vi "Standard Engine.vi"(8 "error in":errorcluster, 9 "status notifier":refnum<notifier>, 10 "rt fifo":refnum<k33>, 11 "Engine Data":T1={"Main Tag Data"={"Double"=[], "Single"=[], "I64"=[], "I32"=[], "I16"=[], "I8"=[], "U64"=[], "U32"=[], "U16"=[], "U8"=[], "Boolean"=[], "String"=[], "Array of Double"=[], "Array of Single"=[], "Array of I64"=[], "Array of I32"=[], "Array of I16"=[], "Array of I8"=[], "Array of U64"=[], "Array of U32"=[], "Array of U16"=[], "Array of U8"=[], "Array of Boolean"=[], "Array of String"=[]}, "Module Info"={"Tag Bus Modules"=[], "Input Method Indices"=[], "Process Method Indices"=[], "Output Method Indices"=[], "Input Transfer Specifications"=[], "Parameter Transfer Specifications"=[], "Result Transfer Specifications"=[], "Output Transfer Specifications"=[], "Module Errors"=[], "UID"=""}, "Safe State?"=FALSE, "engine timing source"=refnum, "Processor"=-2, "Priority"=1, "dT"=0}) -> (0 "error out":errorcluster)   [LabVIEW 2013, in "synchronous engine runtime.lvclass"]
uses:
  synchronous engine runtime.lvclass
  Engine Data.ctl
  <vilib>/NI/Module Timing Source/timing source/TBM timing source.lvclass
  <vilib>/NI/Tag Bus/table/data table.ctl
  Module Execution Info.ctl
  <vilib>/NI/Tag Bus Module Framework/runtime/TBM module execution interface.lvclass
  Data Table with Transfer Spec.ctl
  <vilib>/NI/Tag Bus/table/transfer specification.ctl
  <vilib>/NI/Tag Bus/tag/Data Type.ctl
  Commands.ctl
  notifier.ctl
  Engine Runtime/Execution States.ctl
  <vilib>/Platform/TimedLoop/XDataNode/timing_clust.ctl
  <vilib>/Platform/TimedLoop/XDataNode/nitl_modes.ctl
  <vilib>/Platform/TimedLoop/XDataNode/wakeup.ctl
  <vilib>/NI/Tag Bus/table/transfer table data.vi
  <vilib>/Platform/TimedLoop/XDataNode/XDataNode.xnode
  Engine Runtime/Engine Runtime Interface.lvclass
  <vilib>/Platform/TimedLoop/XDataNode/XDNodeRunTimeDep.lvlib
  <vilib>/NI/Tag Bus/table/data table.lvlib
  <vilib>/NI/Tag Bus/tag/tag descriptor.lvclass
panel:
  out "iterations":i32
  in  "Network Address":string="10.1.128.117"
  in  "send trace?":bool
  out "loop period (ms)":u32
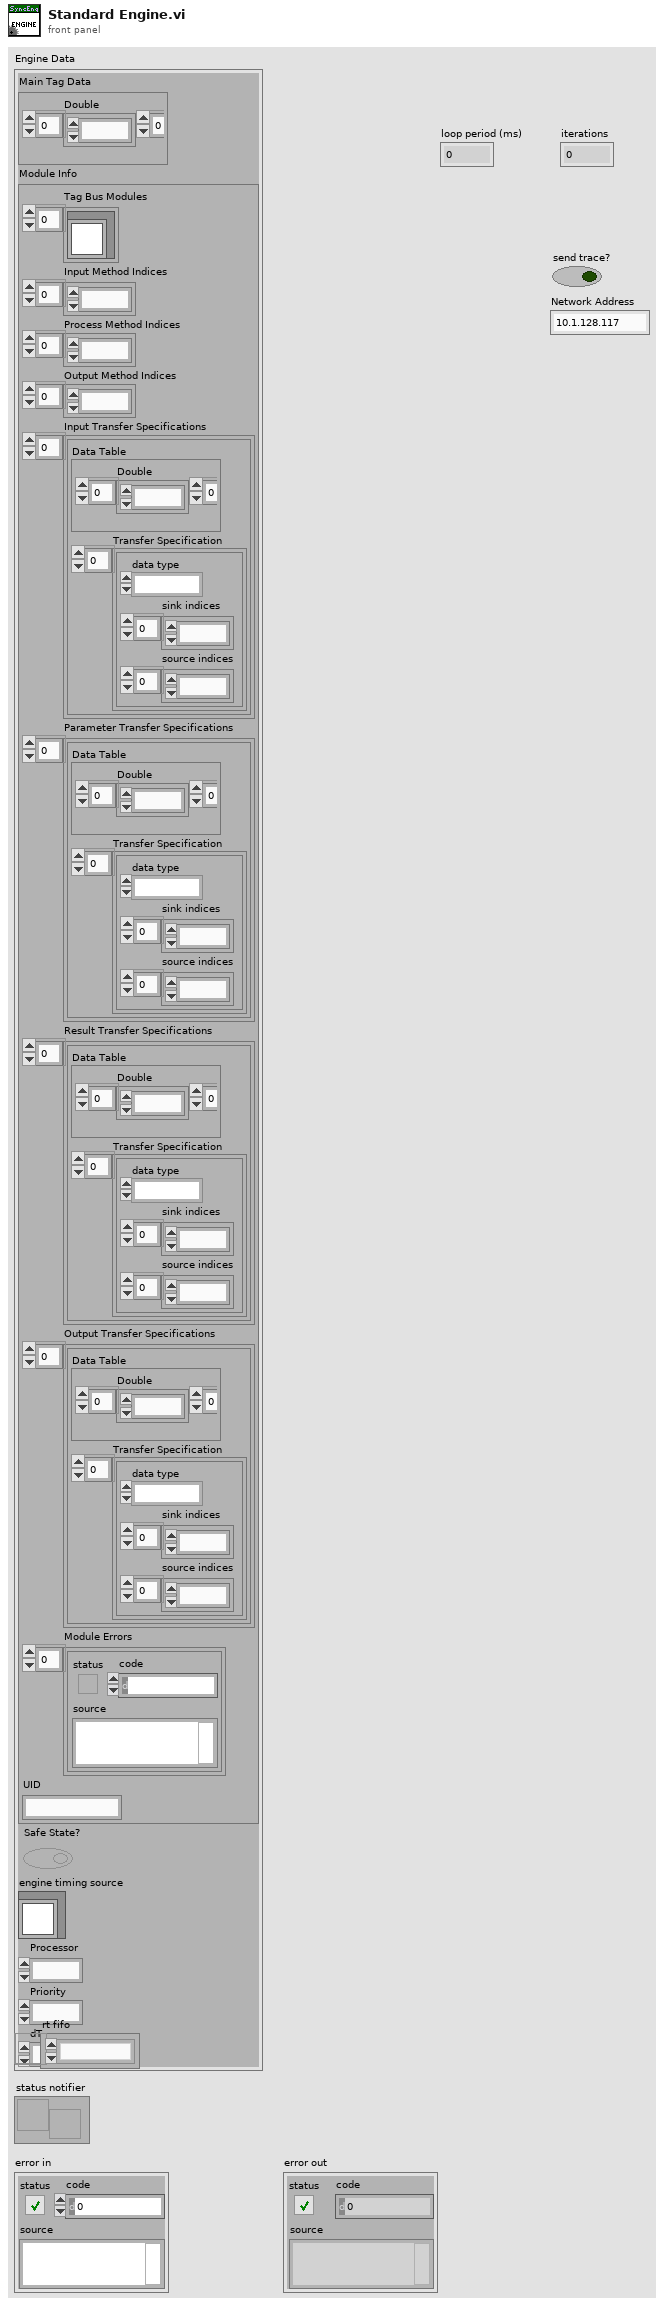
[diagram p1: front panel]
types:
  T1 = typedef "synchronous engine runtime.lvclass/Engine Data.ctl" = cluster{"Main Tag Data":T2, "Module Info":T3, "Safe State?":bool, "engine timing source":refnum<class "TBM timing source.lvclass">, "Processor":i32, "Priority":i32, "dT":u32}
  T2 = typedef "tag bus.lvlib/data table.lvlib/data table.ctl" = cluster{"Double":dbl[], "Single":sgl[], "I64":i64[], "I32":i32[], "I16":i16[], "I8":i8[], "U64":u64[], "U32":u32[], "U16":u16[], "U8":u8[], "Boolean":bool[], "String":string[], "Array of Double":cluster{"DBL Array":dbl[]}[], "Array of Single":cluster{"SGL Array":sgl[]}[], "Array of I64":cluster{"I64 Array":i64[]}[], "Array of I32":cluster{"I32 Array":i32[]}[], "Array of I16":cluster{"I16 Array":i16[]}[], "Array of I8":cluster{"I8 Array":i8[]}[], "Array of U64":cluster{"U64 Array":u64[]}[], "Array of U32":cluster{"U32 Array":u32[]}[], "Array of U16":cluster{"U16 Array":u16[]}[], "Array of U8":cluster{"U8 Array":u8[]}[], "Array of Boolean":cluster{"Boolean Array":bool[]}[], "Array of String":cluster{"String Array":string[]}[]}
  T3 = typedef "synchronous engine runtime.lvclass/Module Execution Info.ctl" = cluster{"Tag Bus Modules":refnum<class "TBM module execution interface.lvclass">[], "Input Method Indices":i32[], "Process Method Indices":i32[], "Output Method Indices":i32[], "Input Transfer Specifications":T4[], "Parameter Transfer Specifications":T4[], "Result Transfer Specifications":T4[], "Output Transfer Specifications":T4[], "Module Errors":errorcluster[], "UID":string}
  T4 = typedef "synchronous engine runtime.lvclass/Data Table with Transfer Spec.ctl" = cluster{"Data Table":T2, "Transfer Specification":T5[]}
  T5 = typedef "tag bus.lvlib/data table.lvlib/transfer specification.ctl" = cluster{"data type":T6, "sink indices":i32[], "source indices":i32[]}
  T6 = typedef "tag bus.lvlib/tag descriptor.lvclass/Data Type.ctl" = enum16{"Double", "Single", "I64", "I32", "I16", "I8", "U64", "U32", "U16", "U8", "Boolean", "String", "Array of Double", "Array of Single", "Array of I64", "Array of I32", "Array of I16", "Array of I8", "Array of U64", "Array of U32", "Array of U16", "Array of U8", "Array of Boolean", "Array of String"}
  T7 = typedef "Engine Runtime Interface.lvclass/Execution States.ctl" = enum16{"Initializing", "Paused (Initialized)", "Running", "Set Safe Outputs", "Uninitializing", "Stopped (Uninitialized)", "Error (Uninitialized)", "Safe State (Uninitialized)", "Closed"}
  T8 = typedef "synchronous engine runtime.lvclass/notifier.ctl" = cluster{"Engine State":T7, "error constant":errorcluster}
  T9 = typedef "synchronous engine runtime.lvclass/Commands.ctl" = enum16{"Start", "Pause", "Safe State", "Normal", "Stop", "Shutdown"}
  T10 = typedef "XDNodeRunTimeDep.lvlib/timing_clust.ctl" = cluster{"Expected End [f-1]":u64, "Actual End [f-1]":u64, "Finished Late? [f-1]":bool, "Expected End [i-1]":u64, "Actual End [i-1]":u64, "Finished Late? [i-1]":bool, "Expected Start [i]":u64, "Actual Start [i]":u64, "Expected Start [f]":u64, "Actual Start [f]":u64, "Source Name":string, "Structure Name":string, "Period":i64, "Deadline":i64, "Offset":i64, "Start":i64, "Priority":i32, "Timeout":i32, "Mode":T11, "Wakeup Reason":T12, "Error":errorcluster, "Source Type":string, "Secondary Source Type":string, "Global End Time":u64, "Global Start Time":u64, "Frame Duration":u64, "Iteration Duration":u64, "Assigned CPU":i32, "I/O Scan Engine Mode":u32}
  T11 = typedef "XDNodeRunTimeDep.lvlib/nitl_modes.ctl" = enum32{"No Change", "Process missed periods, maintain original phase", "Discard missed periods, maintain original phase", "Process missed periods, ignore original phase", "Discard missed periods, ignore original phase"}
  T12 = typedef "XDNodeRunTimeDep.lvlib/wakeup.ctl" = enum32{"Normal", "Aborted", "Asynchronous wakeup", "Timing source error", "Timed loop error", "Timeout"}
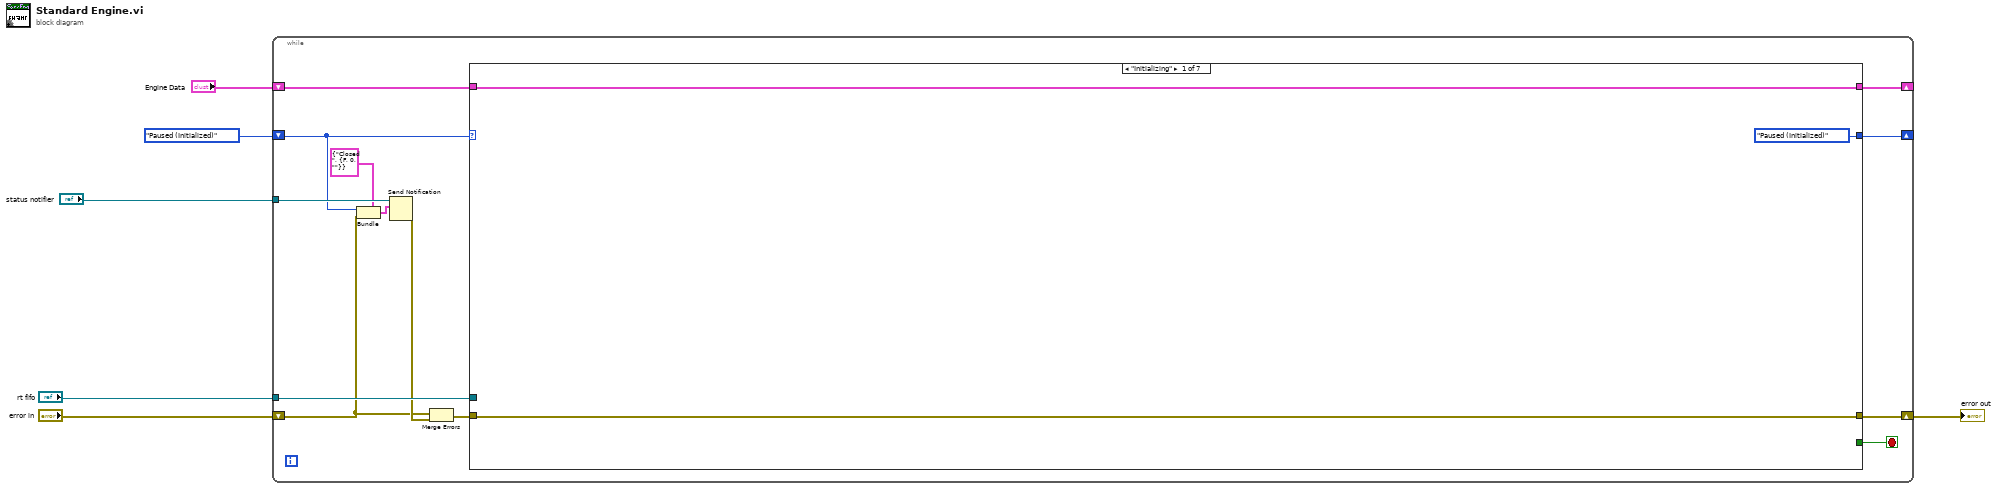
[diagram p0: block diagram]
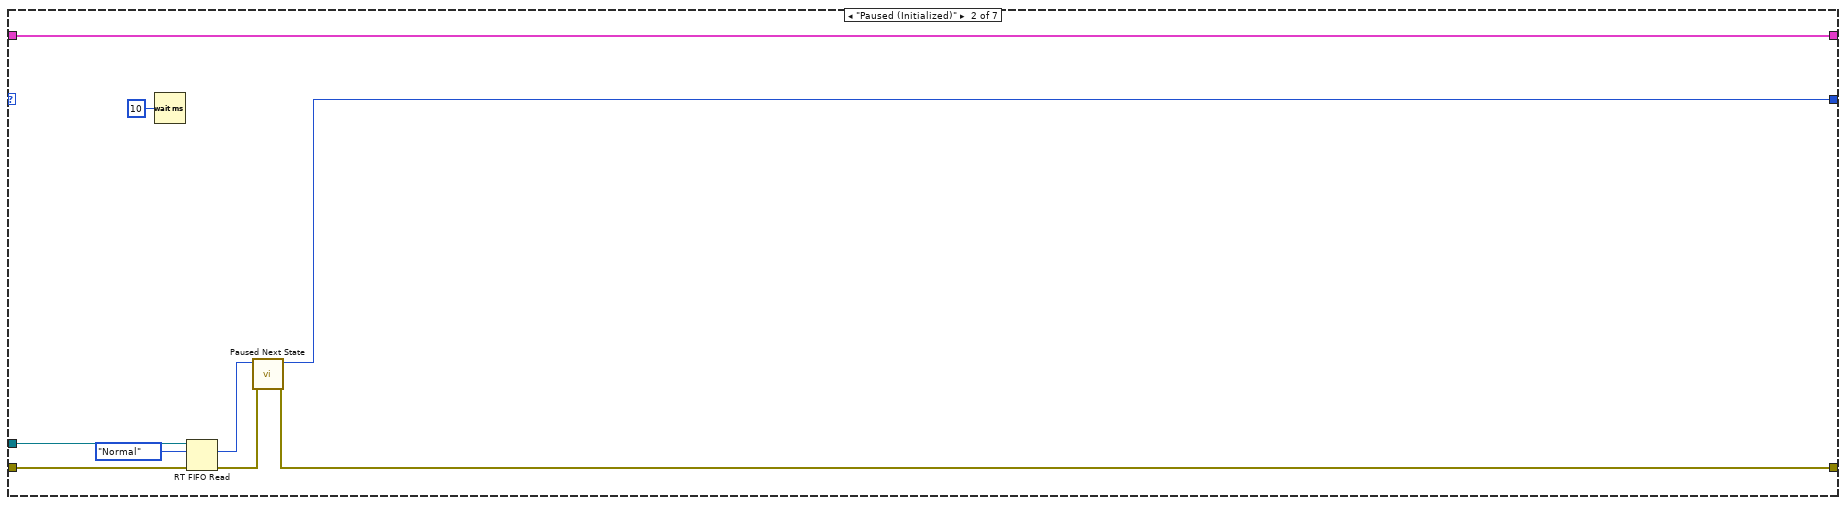
[diagram p2: hidden frame]
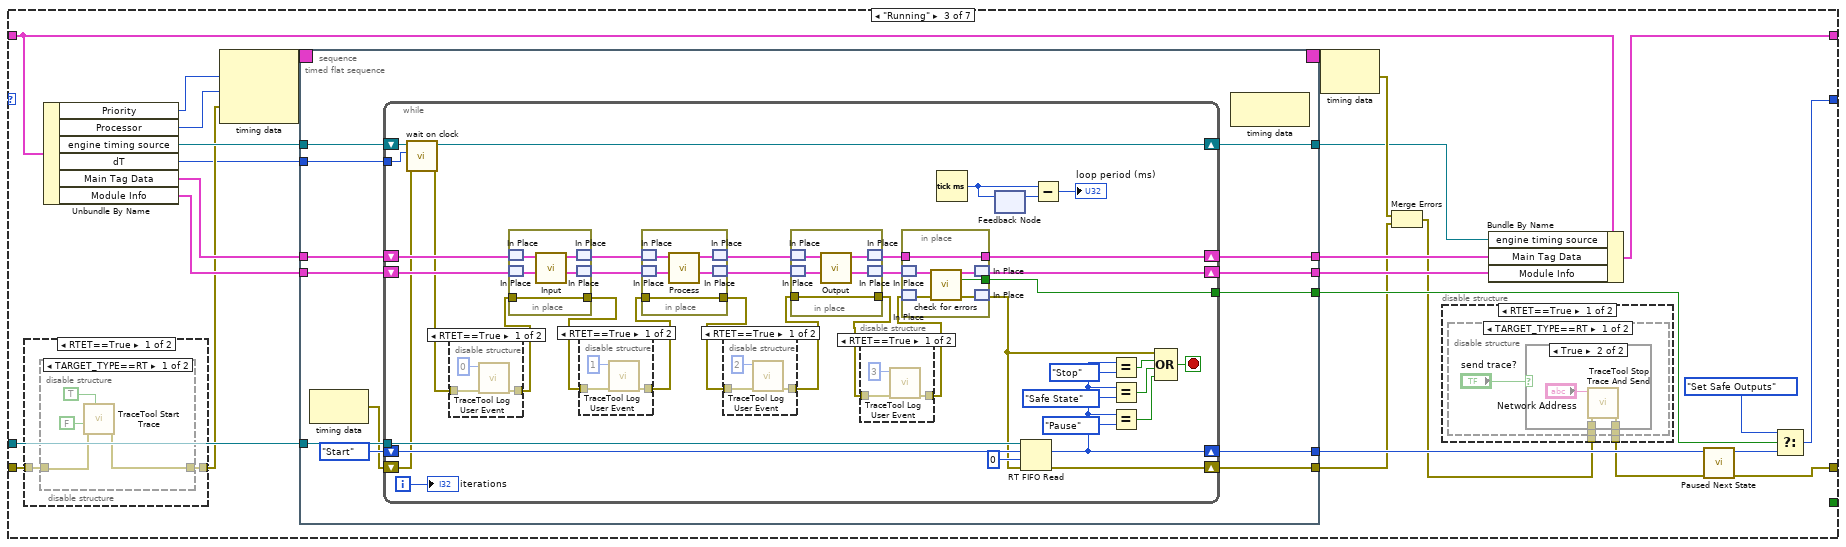
[diagram p3: hidden frame]
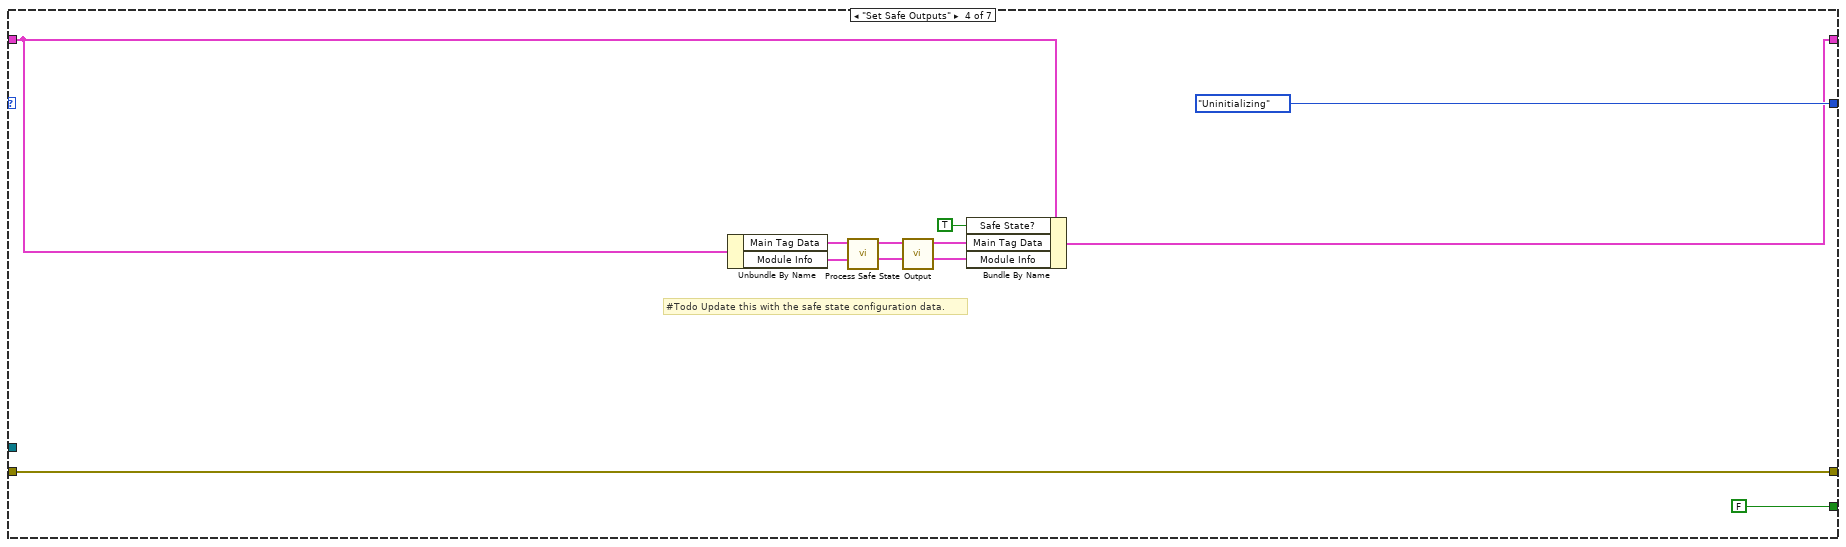
[diagram p13: hidden frame]
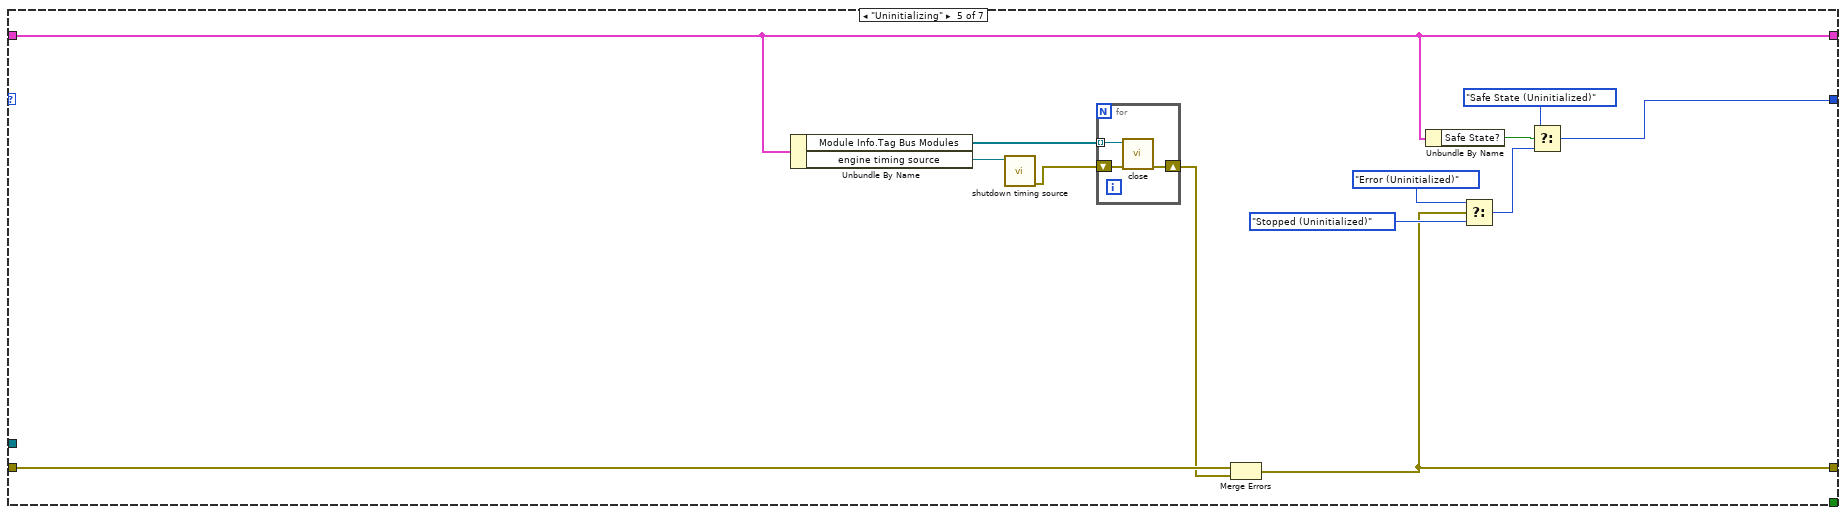
[diagram p14: hidden frame]
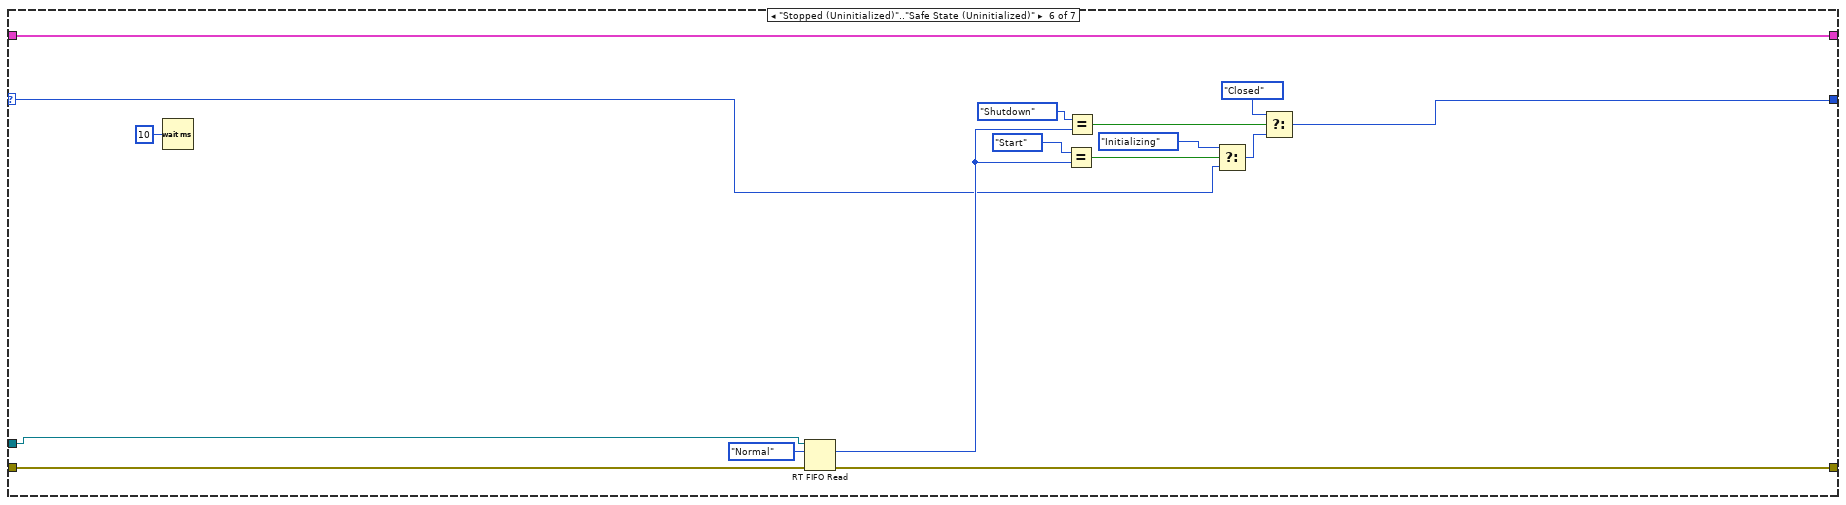
[diagram p15: hidden frame]
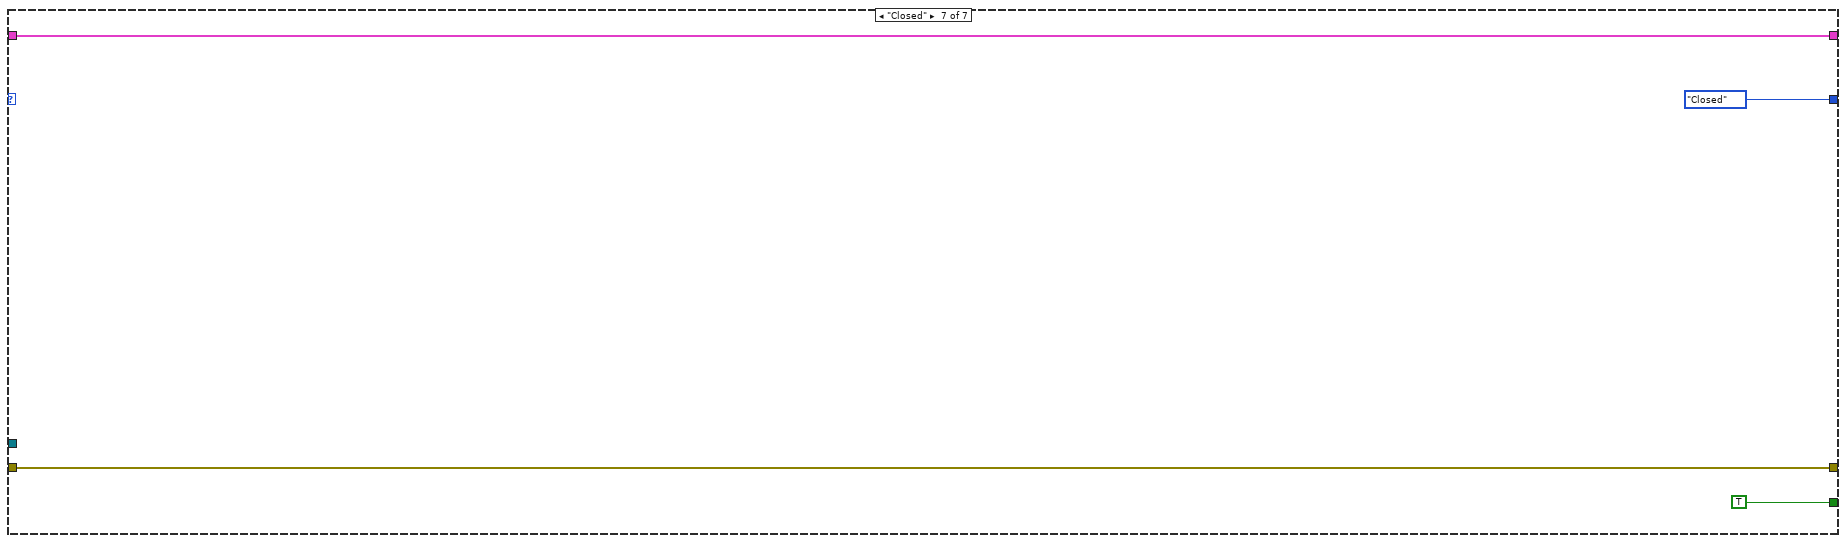
[diagram p16: hidden frame]
diagram:
  n1 = while {
    shift-right: [w16] -> _
    shift-left: Execution_States."Paused (Initialized)" ("States") -> [w10]
    shift-right: [w17] -> _
    shift-left: "Engine Data" -> [w19]
    shift-right: [w18] -> w5
    shift-left: "error in" -> [w7]
    tunnel: "rt fifo" -> [w15]
    tunnel: "status notifier" -> [w13]
    stop <- w14 stop-if-true
    n2 = Bundle(cluster=T8 {"Engine State"=enum."Closed", "error constant"={"status"=FALSE, "code"=0, "source"=""}} ("notification"), "Engine State"=w10, "error constant"=w7) -> (w9:T8)
    n3 = Send Notification(notification=w9, notifier=w13) -> (error out=w12:errorcluster)  [unwired: 1 in, 1 out]
    n4 = Merge Errors(w7, w12) -> (w8:errorcluster)
    n5 = case shown="\"Initializing\"" w10 {
      selector: w10 -> [_ _ _ _ _ w217 _]
      tunnel: w19 -> [w22 w31 w33 w191 w201 w216 w233]
      tunnel: w8 -> [w21 w30 w45 w199 w205 w219 w235]
      tunnel: [w21 w24 w50 w199 w203 w226 w235] -> w18
      tunnel: [w22 w31 w34 w190 w201 w216 w233] -> w17
      tunnel: [Execution_States."Paused (Initialized)" ("States") w28 w46 Execution_States."Uninitializing" ("States") w207 w228 Execution_States."Closed" ("States")] -> w16
      tunnel: w15 -> [_ w23 w57 _ _ w218 _]
      tunnel: [_ _ _ FALSE _ _ TRUE] -> w14
      frame "Initializing" {
      }
      frame "Paused (Initialized)" {
        n6 = Wait (ms)(milliseconds to wait=u32 10) -> ()  [unwired: 1 out]
        n7 = RT FIFO Read(0:w23, 1:Commands."Normal" ("Commands"), 3:w30) -> (9:w27:T9, 11:w26:errorcluster)  [unwired: 1 in, 3 out]
        n8 = call "Paused Next State.vi"("error in"=w26, "Command"=w27) -> ("error out"=w24:errorcluster, "State"=w28:T7)  [unwired: 8 in]
      }
      frame "Running" {
        n9 = disable-structure shown="RTET==True" {
          disable-tunnel: w45 -> [w181 w187]
          disable-tunnel: [w180 w187] -> w40
          frame condition #0 {
            n10 = disable-structure shown="TARGET_TYPE==RT" {
              disable-tunnel: w181 -> [w182 w186]
              disable-tunnel: [w183 w186] -> w180
              frame condition #0 {
                n11 = call <vilib>:"TraceTool Start Trace.vi"("Detailed Tracing? (F)"=TRUE, "error in (no error)"=w182, "VI Tracing? (T)"=FALSE) -> ("error out"=w183:errorcluster)  [unwired: 7 in, 1 out]
              }
              frame condition #1 (active) {
              }
            }
          }
          frame condition #1 (active) {
          }
        }
        n12 = Unbundle By Name(w33) -> ("Priority"=w35:i32, "Processor"=w36:i32, "engine timing source"=w41:refnum<class "TBM timing source.lvclass">, "dT"=w32:u32, "Main Tag Data"=w56:T2, "Module Info"=w55:T3)
        n13 = node-c288(w35, w36, w40) -> (w38:T10)
        n14 = timed-sequence {
          timing: w38 -> [_]
          timing-out: [_] -> w37
          tunnel: w57 -> [w68]
          tunnel: w56 -> [w67]
          tunnel: w55 -> [w66]
          tunnel: [w65] -> w54
          tunnel: [w64] -> w53
          tunnel: [w63] -> w52
          tunnel: [w62] -> w48
          tunnel: [w61] -> w44
          tunnel: w41 -> [w59]
          tunnel: [w60] -> w39
          tunnel: w32 -> [w58]
          n15 = timed-flat-sequence {
            tunnel: w68 -> [w81]
            tunnel: w67 -> [w79]
            tunnel: w66 -> [w78]
            tunnel: [w77] -> w65
            tunnel: [w76] -> w64
            tunnel: [w75] -> w63
            tunnel: [w74] -> w62
            tunnel: [w72] -> w61
            tunnel: [w71] -> w60
            tunnel: w59 -> [w70]
            tunnel: w58 -> [w69]
            n16 = node-c288() -> (w73:errorcluster)  [unwired: 1 in]
            n17 = while {
              tunnel: w81 -> [w104]
              shift-right: [w112] -> w75
              shift-left: Commands."Start" ("Commands") -> [w124]
              shift-right: [w101] -> w77
              shift-left: w79 -> [w122]
              shift-right: [w116] -> w76
              shift-left: w78 -> [w121]
              tunnel: [w99] -> w74
              shift-right: [w103] -> w72
              shift-left: w73 -> [w88]
              shift-right: [w86] -> w71
              shift-left: w70 -> [w89]
              tunnel: w69 -> [w85]
              i -> [w98]
              stop <- w105 stop-if-true
              n18 = call-dynamic "wait on clock.vi"("error in"=w88, "dt"=w85, "timing source in"=w89) -> ("error out"=w87:errorcluster, "timing source out"=w86:refnum<class "TBM timing source.lvclass">)  [unwired: 6 in, 1 out]
              n19 = disable-structure shown="RTET==True" {
                disable-tunnel: w87 -> [w139 w140]
                disable-tunnel: [w138 w140] -> w96
                frame condition #0 {
                  n20 = call <vilib>:"TraceTool Log User Event.vi"("error in (no error)"=w139, "Event ID (0-255)"=u32 0) -> ("error out"=w138:errorcluster)  [unwired: 9 in]
                }
                frame condition #1 (active) {
                }
              }
              n21 = in-place {
                in-place-border: w96 -> [w161]
                in-place-border: [w161] -> w95
                n22 = in-place-match #1(w122) -> (w160:T2)
                n23 = in-place-match #2(w121) -> (w157:T3)
                n24 = call "Input.vi"("Module Info In"=w157, "Engine Tags In"=w160) -> ("Module Info Out"=w158:T3, "Engine Tags Out"=w159:T2)  [unwired: 8 in]
                n25 = in-place-match #1(w159) -> (w120:T2)
                n26 = in-place-match #2(w158) -> (w119:T3)
              }
              n27 = disable-structure shown="RTET==True" {
                disable-tunnel: w95 -> [w135 w136]
                disable-tunnel: [w134 w136] -> w94
                frame condition #0 {
                  n28 = call <vilib>:"TraceTool Log User Event.vi"("error in (no error)"=w135, "Event ID (0-255)"=u32 1) -> ("error out"=w134:errorcluster)  [unwired: 9 in]
                }
                frame condition #1 (active) {
                }
              }
              n29 = in-place {
                in-place-border: w94 -> [w156]
                in-place-border: [w156] -> w93
                n30 = in-place-match #3(w120) -> (w155:T2)
                n31 = in-place-match #4(w119) -> (w152:T3)
                n32 = call "Process.vi"("Module Info In"=w152, "Engine Tags In"=w155) -> ("Module Info Out"=w153:T3, "Engine Tags Out"=w154:T2)  [unwired: 8 in]
                n33 = in-place-match #3(w154) -> (w97:T2)
                n34 = in-place-match #4(w153) -> (w118:T3)
              }
              n35 = disable-structure shown="RTET==True" {
                disable-tunnel: w93 -> [w131 w132]
                disable-tunnel: [w130 w132] -> w92
                frame condition #0 {
                  n36 = call <vilib>:"TraceTool Log User Event.vi"("error in (no error)"=w131, "Event ID (0-255)"=u32 2) -> ("error out"=w130:errorcluster)  [unwired: 9 in]
                }
                frame condition #1 (active) {
                }
              }
              n37 = in-place {
                in-place-border: w92 -> [w151]
                in-place-border: [w151] -> w91
                n38 = in-place-match #5(w97) -> (w150:T2)
                n39 = in-place-match #6(w118) -> (w149:T3)
                n40 = call "Output.vi"("Module Info In"=w149, "Engine Tags In"=w150) -> ("Module Info Out"=w148:T3, "Engine Tags Out"=w147:T2)  [unwired: 8 in]
                n41 = in-place-match #5(w147) -> (w100:T2)
                n42 = in-place-match #6(w148) -> (w117:T3)
              }
              n43 = disable-structure shown="RTET==True" {
                disable-tunnel: w91 -> [w127 w128]
                disable-tunnel: [w126 w128] -> w90
                frame condition #0 {
                  n44 = call <vilib>:"TraceTool Log User Event.vi"("error in (no error)"=w127, "Event ID (0-255)"=u32 3) -> ("error out"=w126:errorcluster)  [unwired: 9 in]
                }
                frame condition #1 (active) {
                }
              }
              n45 = in-place {
                in-place-border: [w146] -> w101
                in-place-border: w100 -> [w146]
                in-place-border: [w141] -> w99
                n46 = in-place-match #7(w117) -> (w144:T3)
                n47 = in-place-match #8(w90) -> (w142:errorcluster)
                n48 = call "check for errors.vi"("error in"=w142, "Module Info in"=w144) -> ("error out"=w143:errorcluster, "safe state"=w141:bool, "Module Info out"=w145:T3)  [unwired: 7 in]
                n49 = in-place-match #7(w145) -> (w116:T3)
                n50 = in-place-match #8(w143) -> (w102:errorcluster)
              }
              n51 = Tick Count (ms)() -> (millisecond timer value=w115:u32)
              n52 = feedback-in #9(w115) -> ()
              n53 = feedback #9() -> (w114:u32)  [unwired: 1 in]
              n54 = RT FIFO Read(0:w104, 1:w124, 2:0 ("timeout in ms (0)"), 3:w102) -> (9:w112:T9, 11:w103:errorcluster)  [unwired: 3 out]
              n55 = Subtract(x=w115, y=w114) -> (x-y=→"loop period (ms)":u32)
              n56 = Equal?(x=w112, y=Commands."Stop") -> (x = y?=w108:bool)
              n57 = Equal?(x=w112, y=Commands."Safe State") -> (x = y?=w107:bool)
              n58 = Equal?(x=w112, y=Commands."Pause") -> (x = y?=w106:bool)
              n59 = Compound Arithmetic op=OR(w102, w108, w107, w106) -> (w105:bool)
              "iterations" <- w98
            }
            n60 = node-c288() -> ()  [unwired: 1 in, 1 out]
          }
        }
        n61 = node-c288(w37) -> (w42:errorcluster)
        n62 = Merge Errors(w42, w44) -> (w43:errorcluster)
        n63 = disable-structure shown="RTET==True" {
          disable-tunnel: [w170 w179] -> w51
          disable-tunnel: w43 -> [w169 w179]
          frame condition #0 {
            n64 = disable-structure shown="TARGET_TYPE==RT" {
              disable-tunnel: [w173 w178] -> w170
              disable-tunnel: w169 -> [w172 w178]
              frame condition #0 {
                n65 = case shown="True" "send trace?" {
                  tunnel: [w174 w177] -> w173
                  tunnel: w172 -> [w174 w176]
                  frame False {
                  }
                  frame True {
                    n66 = call <vilib>:"TraceTool Stop Trace And Send.vi"("error in (no error)"=w176, "Trace Host Network Address"="Network Address") -> ("error out"=w177:errorcluster)  [unwired: 9 in]
                  }
                }
              }
              frame condition #1 (active) {
              }
            }
          }
          frame condition #1 (active) {
          }
        }
        n67 = Bundle By Name(cluster=w33, "engine timing source"=w39, "Main Tag Data"=w54, "Module Info"=w53) -> (w34:T1)
        n68 = call "Paused Next State.vi"("error in"=w51, "Command"=w52) -> ("error out"=w50:errorcluster, "State"=w49:T7)  [unwired: 8 in]
        n69 = Select(t=Execution_States."Set Safe Outputs", s=w48, f=w49) -> (s? t:f=w46:T7)
      }
      frame "Set Safe Outputs" {
        # "#Todo Update this with the safe state configuration data."
        n70 = Unbundle By Name(w191) -> ("Main Tag Data"=w189:T2, "Module Info"=w188:T3)
        n71 = call "Process Safe State.vi"("Module Info In"=w188, "Engine Tags In"=w189) -> ("Module Info Out"=w194:T3, "Engine Tags Out"=w195:T2)  [unwired: 8 in]
        n72 = call "Output.vi"("Module Info In"=w194, "Engine Tags In"=w195) -> ("Module Info Out"=w192:T3, "Engine Tags Out"=w193:T2)  [unwired: 8 in]
        n73 = Bundle By Name(cluster=w191, "Safe State?"=TRUE, "Main Tag Data"=w193, "Module Info"=w192) -> (w190:T1)
      }
      frame "Uninitializing" {
        n74 = Unbundle By Name(w201) -> ("Module Info.Tag Bus Modules"=w212:refnum<class "TBM module execution interface.lvclass">[], "engine timing source"=w202:refnum<class "TBM timing source.lvclass">)
        n75 = call-dynamic "shutdown timing source.vi"("timing source in"=w202) -> ("error out"=w206:errorcluster)  [unwired: 9 in, 1 out]
        n76 = for {
          tunnel: w212 -> [w213] mode=indexing
          shift-right: [w214] -> w204
          shift-left: w206 -> [w215]
          n77 = call-dynamic "close.vi"("error in"=w215, "module in"=w213) -> ("error out"=w214:errorcluster)  [unwired: 9 in]
        }
        n78 = Merge Errors(w205, w204) -> (w203:errorcluster)
        n79 = Unbundle By Name(w201) -> ("Safe State?"=w200:bool)
        n80 = Select(t=Execution_States."Error (Uninitialized)" ("States"), s=w203, f=Execution_States."Stopped (Uninitialized)" ("States")) -> (s? t:f=w208:T7)
        n81 = Select(t=Execution_States."Safe State (Uninitialized)" ("States"), s=w200, f=w208) -> (s? t:f=w207:T7)
      }
      frame "Stopped (Uninitialized)".."Safe State (Uninitialized)" {
        n82 = Wait (ms)(milliseconds to wait=u32 10) -> ()  [unwired: 1 out]
        n83 = RT FIFO Read(0:w218, 1:Commands."Normal" ("Commands"), 3:w219) -> (9:w231:T9, 11:w226:errorcluster)  [unwired: 1 in, 3 out]
        n84 = Equal?(x=Commands."Start" ("Commands"), y=w231) -> (x = y?=w230:bool)
        n85 = Equal?(x=Commands."Shutdown" ("Commands"), y=w231) -> (x = y?=w225:bool)
        n86 = Select(t=Execution_States."Initializing" ("States"), s=w230, f=w217) -> (s? t:f=w229:T7)
        n87 = Select(t=Execution_States."Closed" ("States"), s=w225, f=w229) -> (s? t:f=w228:T7)
      }
      frame "Closed" {
      }
    }
  }
  "error out" <- w5
